vi "Leftover Merge.vi"(7 "Leftovers":T2(array[cluster]), 10 "Secondary hits":T2(array[cluster]), 11 "Primary hits":T1) -> (2 "Secondary hits out":T2(array[cluster]), 3 "Primary hits out":T1)   [LabVIEW 2016]
uses:
  Global Variables/System info.vi
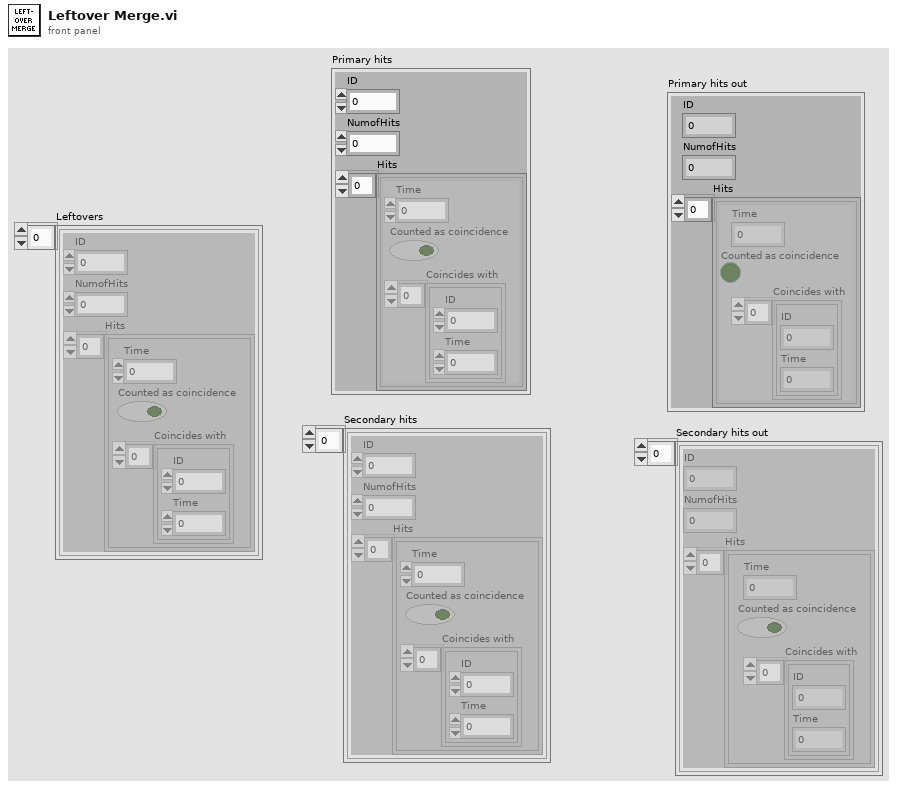
[diagram p1: front panel]
types:
  T1 = cluster{"ID":i8, "NumofHits":i32, "Hits":cluster{"Time":u64, "Counted as coincidence":bool, "Coincides with":cluster{"ID":i8, "Time":u64}[]}[]}
  T2 = cluster{"ID":i8, "NumofHits":i32, "Hits":cluster{"Time":u64, "Counted as coincidence":bool, "Coincides with":cluster{"ID":i8, "Time":u64}[]}[]}[]
  T3 = cluster{"Time":u64, "Counted as coincidence":bool, "Coincides with":cluster{"ID":i8, "Time":u64}[]}[]
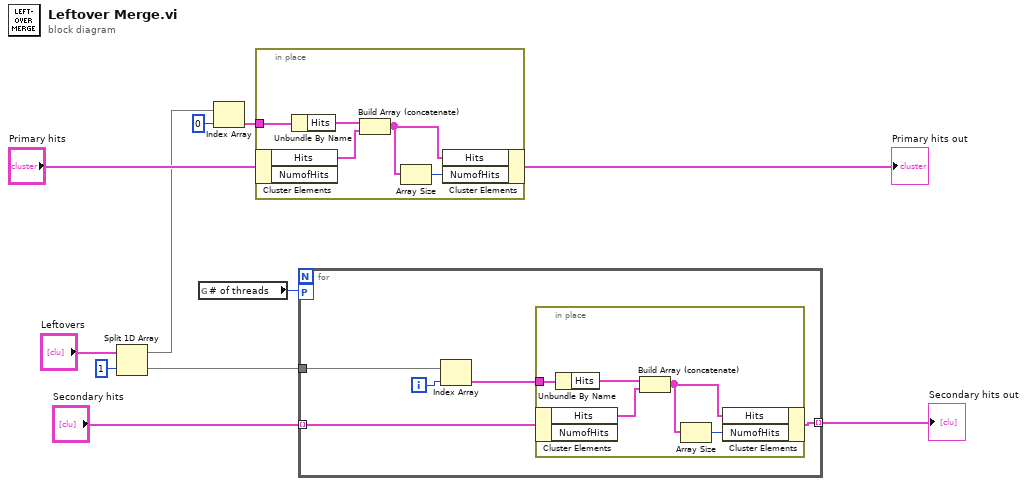
[diagram p0: block diagram]
diagram:
  n1 = Split 1D Array(array="Leftovers", index=1) -> (first subarray=w4:T2, second subarray=w7:T2)
  n2 = global read "System info.vi" "# of threads"() -> (w9:i32)
  n3 = Index Array(array=w4, index=0) -> (element=w2:T1)
  n4 = in-place {
    in-place-border: w2 -> [w16]
    n5 = in-place-cluster #1("Primary hits") -> ("Hits"=w14:T3)  [unwired: 1 out]
    n6 = Unbundle By Name(w16) -> ("Hits"=w15:T3)
    n7 = Build Array (concatenate)(w15, w14) -> (w13:T3)
    n8 = Array Size(array=w13) -> (size(s)=w12:i32)
    n9 = in-place-cluster #1("Hits"=w13, "NumofHits"=w12) -> (→"Primary hits out":T1)
  }
  n10 = for {
    tunnel: "Secondary hits" -> [w21] mode=indexing
    tunnel: w7 -> [w19]
    tunnel: [w20] -> w10 mode=indexing
    workers-P: w9 -> [_]
    i -> [w18]
    n11 = Index Array(array=w19, index=w18) -> (element=w17:T1)
    n12 = in-place {
      in-place-border: w17 -> [w26]
      n13 = in-place-cluster #2(w21) -> ("Hits"=w24:T3)  [unwired: 1 out]
      n14 = Unbundle By Name(w26) -> ("Hits"=w25:T3)
      n15 = Build Array (concatenate)(w25, w24) -> (w23:T3)
      n16 = Array Size(array=w23) -> (size(s)=w22:i32)
      n17 = in-place-cluster #2("Hits"=w23, "NumofHits"=w22) -> (w20:T1)
    }
  }
  "Secondary hits out" <- w10
